vi "Renishaw-XL80_GetLaserMeasurement.vi"(8 "error in (no error)":errorcluster, 11 "Renishaw-XL80 in":refnum<class "Renishaw-XL80.lvclass">) -> (0 "error out":errorcluster, 1 "pStatus":i32(ring) items=["COUNT_OK"=0, "COUNT_ERROR"=1, "COUNT_TPIN_OCCURRED"=2, "COUNT_DATUMED"=4], 2 "GetLaserMeasurement":dbl, 3 "Renishaw-XL80 out":refnum<class "Renishaw-XL80.lvclass">)   [LabVIEW 2024, in "Renishaw-XL80.lvclass"]
doc: "This method retrieves the latest laser reading. The units for this reading depend upon the measurement mode. For linear and straightness modes the reading is in m. For angular the reading is in radians.\n\nDefinition\nHRESULTGetLaserMeasurement( [out] COUNT_STATUS_CODES *pStatus, [out, retval] double *pVal);\nParameters\npStatus\nA variable that will be set to the COUNT_STATUS_CODES.\n\npVal\nA variable that will be set to the laser measurement (in m or in rad).\n\nComments\nThis method will return with an HRESULT of E_FAIL if the client has not previously connected to a DX10 by calling Connect. The method will also return E_FAIL if the DX10 is not responding.\n\nThe property will normally return an HRESULT of S_OK. However, it will return E_POINTER if the client supplies a null pointer for either pVal or pStatus.\n\nIf the DX10 is responding but the ML10 is not responding, then the last received reading will be retrieved.\n\nThe reading is affected by the MeasurementMode, OpticsFactor, Lambda, and MatCompFactor"
uses:
  Renishaw-XL80.lvclass
  Renishaw-XL80.lvclass/Renishaw-XL80.ctl
  D:/A.C.M/Example CSharp_64/bin/Debug/Interop.DX10SDKADAPTORLib.dll
  Example CSharp_64/bin/Debug/Interop.DX10SDKADAPTORLib.dll
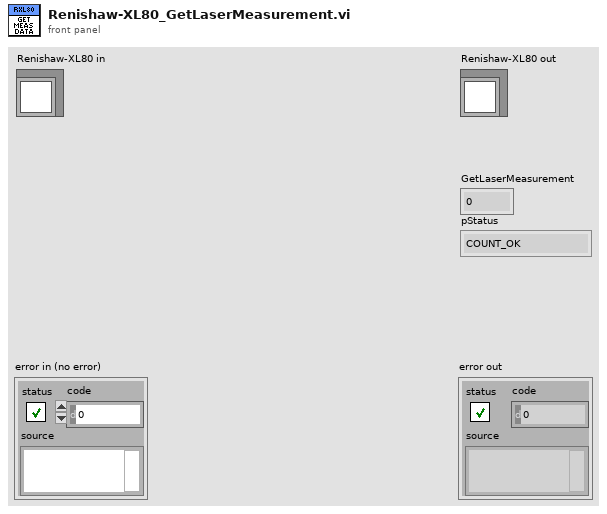
[diagram p1: front panel]
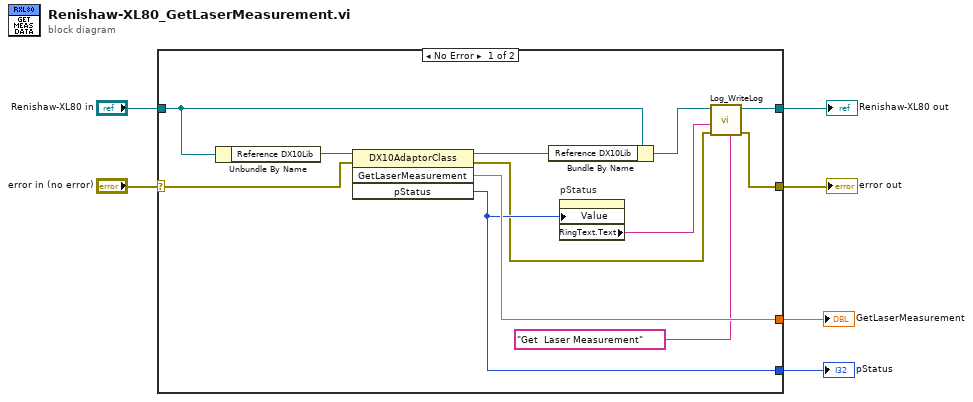
[diagram p0: block diagram]
diagram:
  n1 = case shown="No Error" "error in (no error)" {
    selector: "error in (no error)" -> [w18 w20]
    tunnel: [w9 w20] -> w5
    tunnel: [w12 w19] -> w3
    tunnel: "Renishaw-XL80 in" -> [w17 w19]
    tunnel: [w14 _] -> w2
    tunnel: [w8 _] -> w1
    frame No Error {
      n2 = Unbundle By Name(w17) -> ("Reference DX10Lib"=w15:refnum<k24>)
      n3 = invoke class="DX10AdaptorClass" method="GetLaserMeasurement"(reference=w15, error in=w18) -> (reference out=w16:refnum<k24>, error out=w7:errorcluster, "GetLaserMeasurement"=w14:dbl, "pStatus"=w8:i32)  [unwired: 2 in]
      n4 = Bundle By Name(cluster=w17, "Reference DX10Lib"=w16) -> (w13:refnum<class "Renishaw-XL80.lvclass">)
      n5 = property on="pStatus" class="Ring (strict)"("Value"=w8) -> ("RingText.Text"=w11:string)  [unwired: 2 in, 2 out]
      n6 = call-dynamic "Log_WriteLog.vi"("Additional text"="Get  Laser Measurement", "error in (no error)"=w7, "Response"=w11, "Log in"=w13) -> ("error out"=w9:errorcluster, "Log out"=w12:refnum<class "Renishaw-XL80.lvclass">)  [unwired: 6 in]
    }
    frame Error {
    }
  }
  "error out" <- w5
  "Renishaw-XL80 out" <- w3
  "GetLaserMeasurement" <- w2
  "pStatus" <- w1
